vi "fgt get sensor Status.vi"(8 "error in (no error)":errorcluster, 11 "pressureIndex":u32) -> (0 "error out":errorcluster)   [LabVIEW 2016, in "fgt_SDK.lvlib"]
doc: "Get detailed information of sensor status. This function is ment to be invoked after calling a sensor related function which returns an error code.\n * Retrieved information of last error contains sensor position and a string detail."
uses:
  fgt_SDK.lvlib
  TypeDefs/fgt_STATUS_INFO.ctl
  TypeDefs/fgt_INSTRUMENT_TYPE.ctl
  dlls/fgt_SDK_32.dll
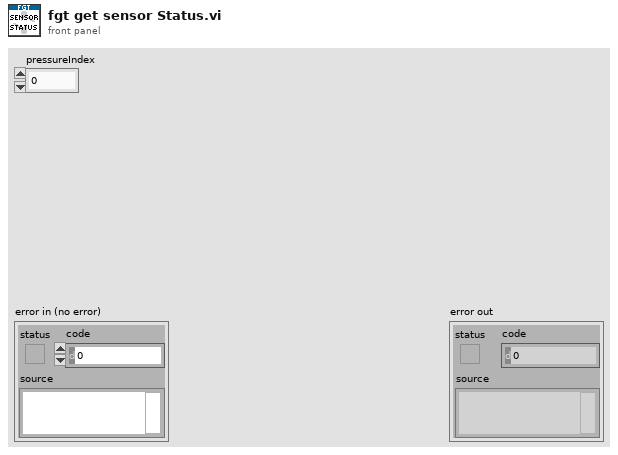
[diagram p1: front panel]
types:
  T1 = typedef "fgt_SDK.lvlib/fgt_STATUS_INFO.ctl" = cluster{"InstrType":T2, "instrSN":u16, "errorCode":u8, "infoCode":u8, "detail":string}
  T2 = typedef "fgt_SDK.lvlib/fgt_INSTRUMENT_TYPE.ctl" = enum32{"None", "MFCS", "MFCS_EZ", "FRP", "LineUP"}
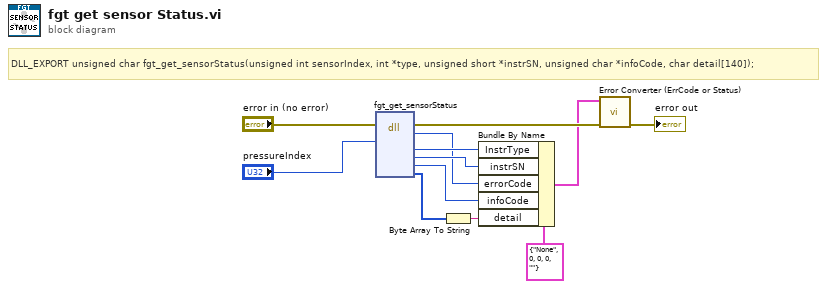
[diagram p0: block diagram]
diagram:
  # "DLL_EXPORT unsigned char fgt_get_sensorStatus(unsigned int sensorIndex, int *type, unsigned short *instrSN, unsigned char *infoCode, char detail[140]);"
  n1 = dll-call lib="PTH2Zabs D\nMes DocumentsDéveloppementFluigentSDKsfgt-sdk-labviewdllsfgt_SDK_*.*" fn="fgt_get_sensorStatus"(error in="error in (no error)", "sensorIndex"="pressureIndex") -> (error out=w10:errorcluster, "return type"=w3:u8, "type"=w6:i32, "instrSN"=w7:u16, "infoCode"=w4:u8, "detail"=w2:i8[])  [unwired: 7 in, 1 out]
  n2 = Byte Array To String(unsigned byte array=w2) -> (string=w1:string)
  n3 = Bundle By Name(cluster=T1 {"InstrType"=enum."None", "instrSN"=0, "errorCode"=0, "infoCode"=0, "detail"=""} ("Cluster"), "InstrType"=w6, "instrSN"=w7, "errorCode"=w3, "infoCode"=w4, "detail"=w1) -> (w5:T1)
  n4 = call "Error Converter (ErrCode or Status).vi"("error in (no error)"=w10, "StatusInfo"=w5) -> ("error out"=→"error out":errorcluster)  [unwired: 9 in]
